vi "Read Dynamic Test Methods.vi"(8 "error in (no error)":errorcluster, 10 "Test Case":string, 11 "Test Case Finder In":refnum<class "Test Finder.lvclass">) -> (0 "error out":errorcluster, 2 "Dynamic Test Methods":map{string, path}(c390), 3 "Test Case Finder Out":refnum<class "Test Finder.lvclass">)   [LabVIEW 2020, in "Test Finder.lvclass"]
uses:
  Test Finder.lvclass
  Test Finder.lvclass/Test Finder.ctl
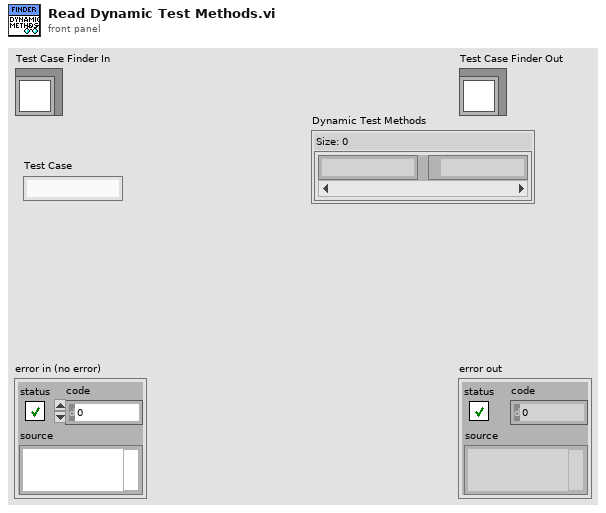
[diagram p1: front panel]
types:
  T1 = map{string, cluster{"Inherited Methods":map{string, path}, "Owned Methods":map{string, path}}}
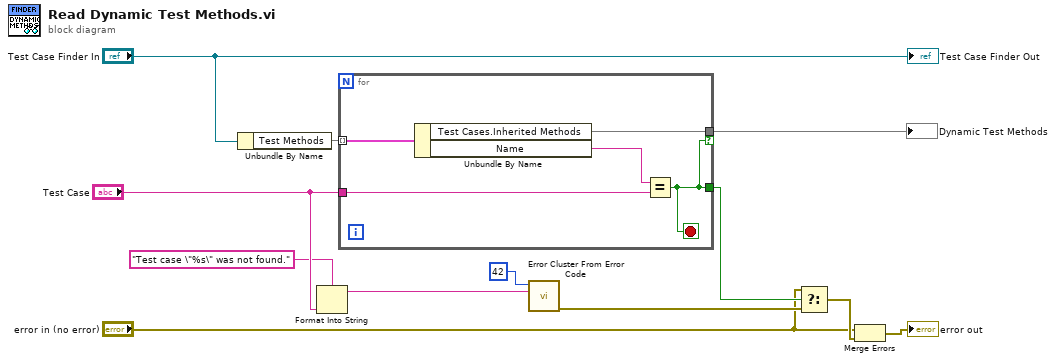
[diagram p0: block diagram]
diagram:
  n1 = Unbundle By Name("Test Case Finder In") -> ("Test Methods"=w11:T1)
  n2 = Format Into String(format string="Test case \"%s\" was not found.", "Test Case") -> (resulting string=w3:string)  [unwired: 2 in, 1 out]
  n3 = for {
    tunnel: w11 -> [w17] mode=indexing
    tunnel: [w14] -> w1 if=w13
    tunnel: "Test Case" -> [w15]
    tunnel: [w13] -> w10
    stop <- w13 stop-if-true
    n4 = Unbundle By Name(w17) -> ("Test Cases.Inherited Methods"=w14:map{string, path}, "Name"=w16:string)
    n5 = Equal?(x=w16, y=w15) -> (x = y?=w13:bool)
  }
  "Dynamic Test Methods" <- w1
  n6 = call <vilib>:"Error Cluster From Error Code.vi"("error message (\"\")"=w3, "error code (0)"=42) -> ("error out"=w7:errorcluster)  [unwired: 7 in]
  n7 = Select(t="error in (no error)", s=w10, f=w7) -> (s? t:f=w8:errorcluster)
  n8 = Merge Errors("error in (no error)", w8) -> (→"error out":errorcluster)
  "Test Case Finder Out" <- "Test Case Finder In"
